vi "Get Loader Map.vi"(8 "error in (no error)":errorcluster, 11 "CIFPluginManager in":refnum<class "CIFPluginManager.lvclass">) -> (0 "error out":errorcluster, 3 "Loader Map":T1)   [LabVIEW 2021, in "CIFPluginManager.lvclass"]
uses:
  CIFPluginManager.lvclass
  typedef/Loader Map.ctl
  typedef/Loaders.ctl
  typedef/Loader Type.ctl
  <vilib>/gRPC/LabVIEW gRPC Library/Shared/grpcId.ctl
  CIFPluginManager.lvclass/CIFPluginManager.ctl
  <vilib>/gRPC/LabVIEW gRPC Library/grpc-lvsupport-release.lvlib
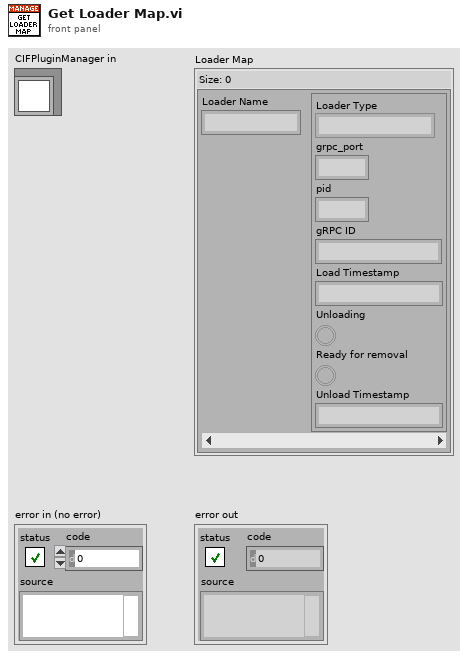
[diagram p1: front panel]
types:
  T1 = typedef "CIFPluginManager.lvclass/Loader Map.ctl" = map{string, T2}
  T2 = typedef "CIFPluginManager.lvclass/Loaders.ctl" = cluster{"Loader Type":T3, "grpc_port":i32, "pid":u32, "gRPC ID":T4, "Load Timestamp":i64, "Unloading":bool, "Ready for removal":bool, "Unload Timestamp":i64}
  T3 = typedef "CIFPluginManager.lvclass/Loader Type.ctl" = enum16{"LabVIEW"}
  T4 = typedef "grpc-lvsupport-release.lvlib/grpcId.ctl" = u64
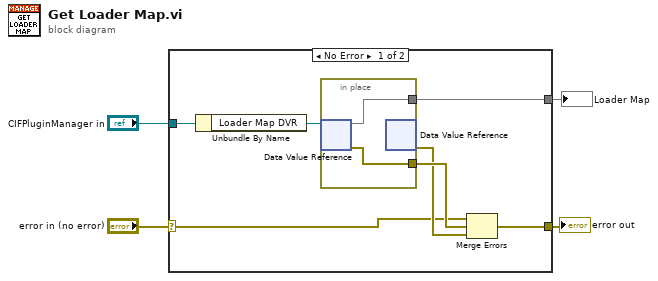
[diagram p0: block diagram]
diagram:
  n1 = case shown="No Error" "error in (no error)" {
    selector: "error in (no error)" -> [w7 w14]
    tunnel: [w6 w14] -> w3
    tunnel: "CIFPluginManager in" -> [w10 _]
    tunnel: [w5 _] -> w1
    frame No Error {
      n2 = Unbundle By Name(w10) -> ("Loader Map DVR"=w11:refnum<data-value>)
      n3 = in-place {
        in-place-border: [w13] -> w5
        in-place-border: [w12] -> w9
        n4 = in-place-dvr #1(w11) -> (w13:T1, w12:errorcluster)
        n5 = in-place-dvr #1() -> (w8:errorcluster)  [unwired: 1 in, 1 out]
      }
      n6 = Merge Errors(w7, w9, w8) -> (w6:errorcluster)
    }
    frame Error {
    }
  }
  "error out" <- w3
  "Loader Map" <- w1
